vi "Configure Reference Calibration Factor.vi"(0 "VISA resource name":refnum<visa-resource-name>, 5 "Power Sensor (0: Power Sensor A)":u16(ring) items=["Power Sensor A", "Power Sensor B"], 7 "Reference Calibration Factor (100.0)":dbl=100.0 format="%.2f", 11 "error in (no error)":errorcluster) -> (4 "VISA resource name out":refnum<visa-resource-name>, 15 "error out":errorcluster)   [LabVIEW 2022 SP3, in "Agilent ENA Series.lvlib"]
doc: "Sets the reference calibration factor (the calibration factor at 50 MHz) for selected power sensor.\n\n<b>Note:</b>\nThis VI is not supported by the E5063A model."
uses:
  <instrlib>/Agilent ENA Series/Agilent ENA Series.lvlib
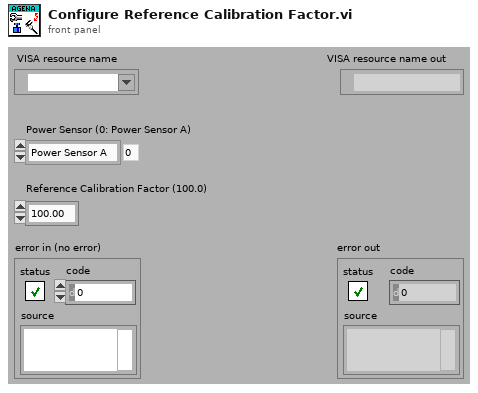
[diagram p1: front panel]
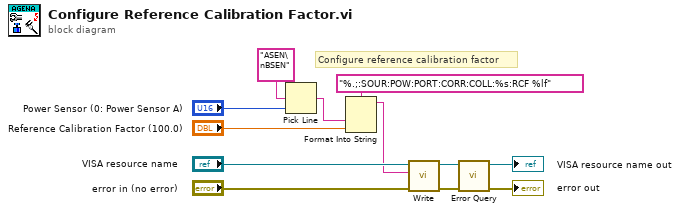
[diagram p0: block diagram]
diagram:
  # "Configure reference calibration factor"
  n1 = Pick Line(multi-line string="ASEN\nBSEN", line index="Power Sensor (0: Power Sensor A)") -> (output string=w8:string)  [unwired: 1 in]
  n2 = Format Into String(format string="%.;:SOUR:POW:PORT:CORR:COLL:%s:RCF %lf", w8, "Reference Calibration Factor (100.0)") -> (resulting string=w5:string)  [unwired: 2 in, 1 out]
  n3 = call <instrlib>:"Write.vi"("error in (no error)"="error in (no error)", "String ()"=w5, "VISA resource name"="VISA resource name") -> ("error out"=w3:errorcluster, "VISA resource name out"=w4:refnum<visa-resource-name>)  [unwired: 6 in, 1 out]
  n4 = call <instrlib>:"Error Query.vi"("error in (no error)"=w3, "VISA resource name"=w4) -> ("error out"=→"error out":errorcluster, "VISA resource name out"=→"VISA resource name out":refnum<visa-resource-name>)  [unwired: 6 in, 2 out]
